vi "ProcessActiveMeasurements.vi"(1 "Active Measurements":T1[](array[typedef])) -> (0 "Measurements":T5)   [LabVIEW 2025]
uses:
  NewCurveDataEventArgs.ctl
  E:/PSCode/PalmSens_SDK/labview/PalmSens/Libraries/PalmSens.Core.Simplified.LabVIEW.dll
  Libraries/PalmSens.Core.Simplified.LabVIEW.dll
  LiveCurveResult.ctl
  MeasurementsResult.ctl
  MeasurementResults.ctl
  CurvesByMeasurement.ctl
  MeasurementInfo.ctl
  CurveInfo.ctl
  MeasurementEventArgs.ctl
  ActiveCurve.ctl
  ActiveMeasurementInfo.ctl
panel:
  out "Processing Completed Event":refnum<user-event>
  out "Active Curve Event":refnum<user-event>
  out "Active Measurement Event":refnum<user-event>
  out "Curves By Measurement":T2
  out "Active Measurement":refnum<k24>
  out "New Curve Values":T8
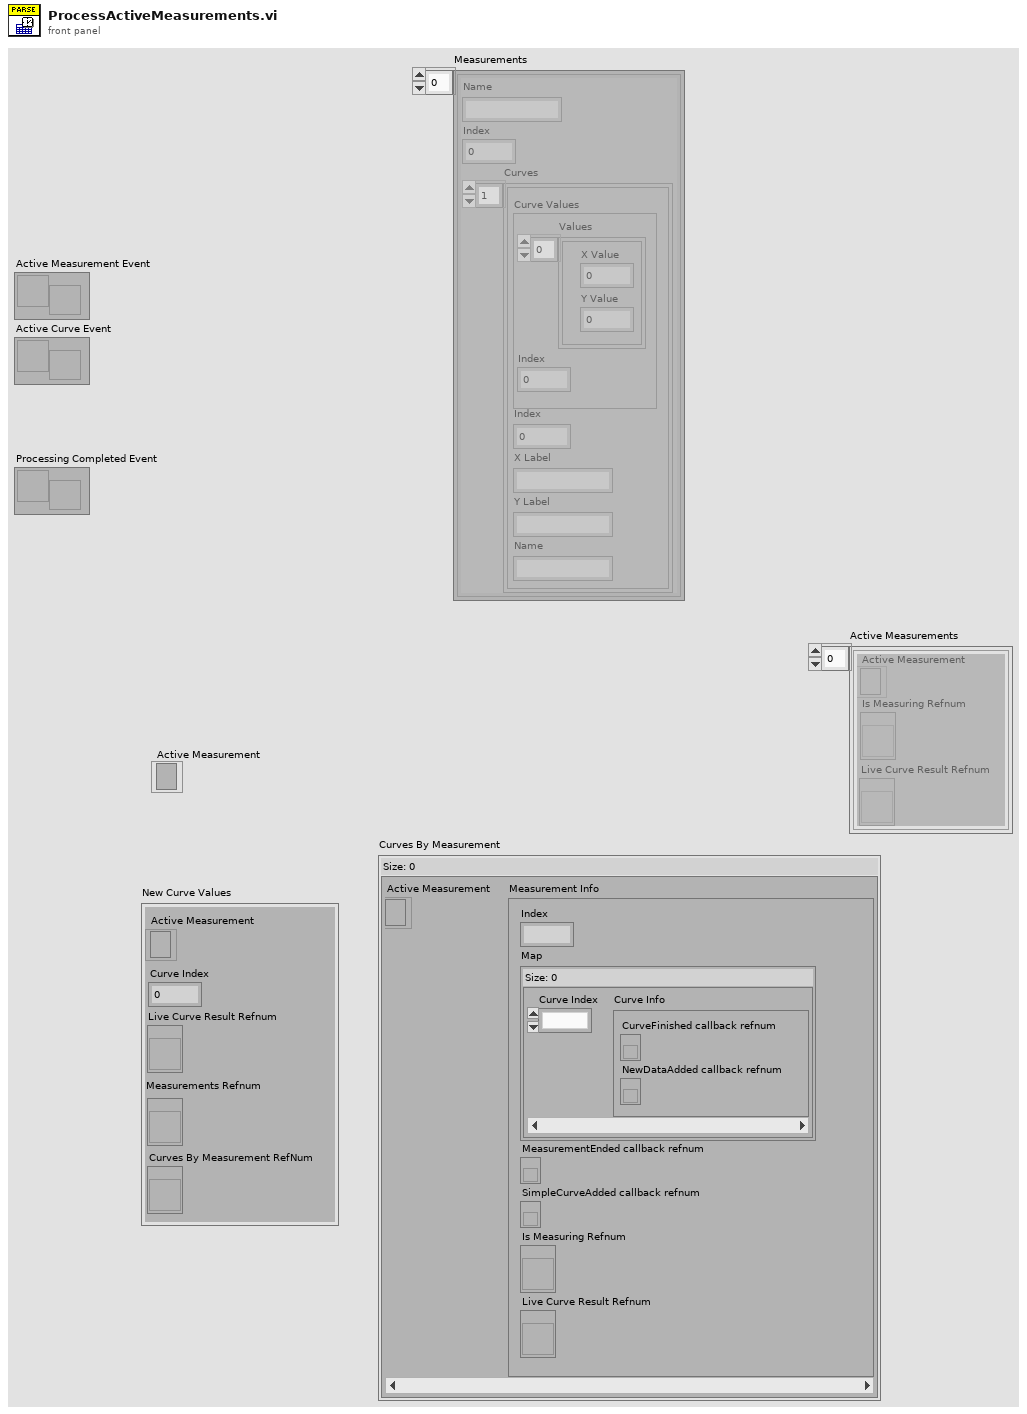
[diagram p1: front panel]
types:
  T1 = typedef "ActiveMeasurementInfo.ctl" = cluster{"Active Measurement":refnum<k24>, "Is Measuring Refnum":refnum<vi>, "Live Curve Result Refnum":refnum<vi>}
  T2 = typedef "CurvesByMeasurement.ctl" = map{refnum<k24>, T3}
  T3 = typedef "MeasurementInfo.ctl" = cluster{"Index":i32, "Is Measuring Refnum":refnum<vi>, "MeasurementEnded callback refnum":refnum<k27>, "SimpleCurveAdded callback refnum":refnum<k27>, "Live Curve Result Refnum":refnum<vi>, "Map":map{i32, T4}}
  T4 = typedef "CurveInfo.ctl" = cluster{"NewDataAdded callback refnum":refnum<k27>, "CurveFinished callback refnum":refnum<k27>}
  T5 = typedef "MeasurementsResult.ctl" = cluster{"Name":string, "Curves":T6, "Index":i32}[]
  T6 = typedef "MeasurementResults.ctl" = T7[]
  T7 = typedef "LiveCurveResult.ctl" = cluster{"X Label":string, "Y Label":string, "Name":string, "Index":i16, "Curve Values":cluster{"Values":cluster{"X Value":dbl, "Y Value":dbl}[], "Index":i16}}
  T8 = typedef "NewCurveDataEventArgs.ctl" = cluster{"Active Measurement":refnum<k24>, "Live Curve Result Refnum":refnum<vi>, "Measurements Refnum":refnum<vi>, "Curves By Measurement RefNum":refnum<vi>, "Curve Index":i32}
  T9 = typedef "ActiveCurve.ctl" = cluster{"Active Measurement":refnum<k24>, "Dispose":bool, "Curve Index":i32}
  T10 = typedef "MeasurementEventArgs.ctl" = cluster{"Active Measurement":refnum<k24>, "Dispose":bool}
  T11 = cluster{"Active Curve":T9, "Active Curve Event":refnum<user-event>}
  T12 = cluster{"Active Measurement":refnum<k24>, "Active Measurement Event":refnum<user-event>}
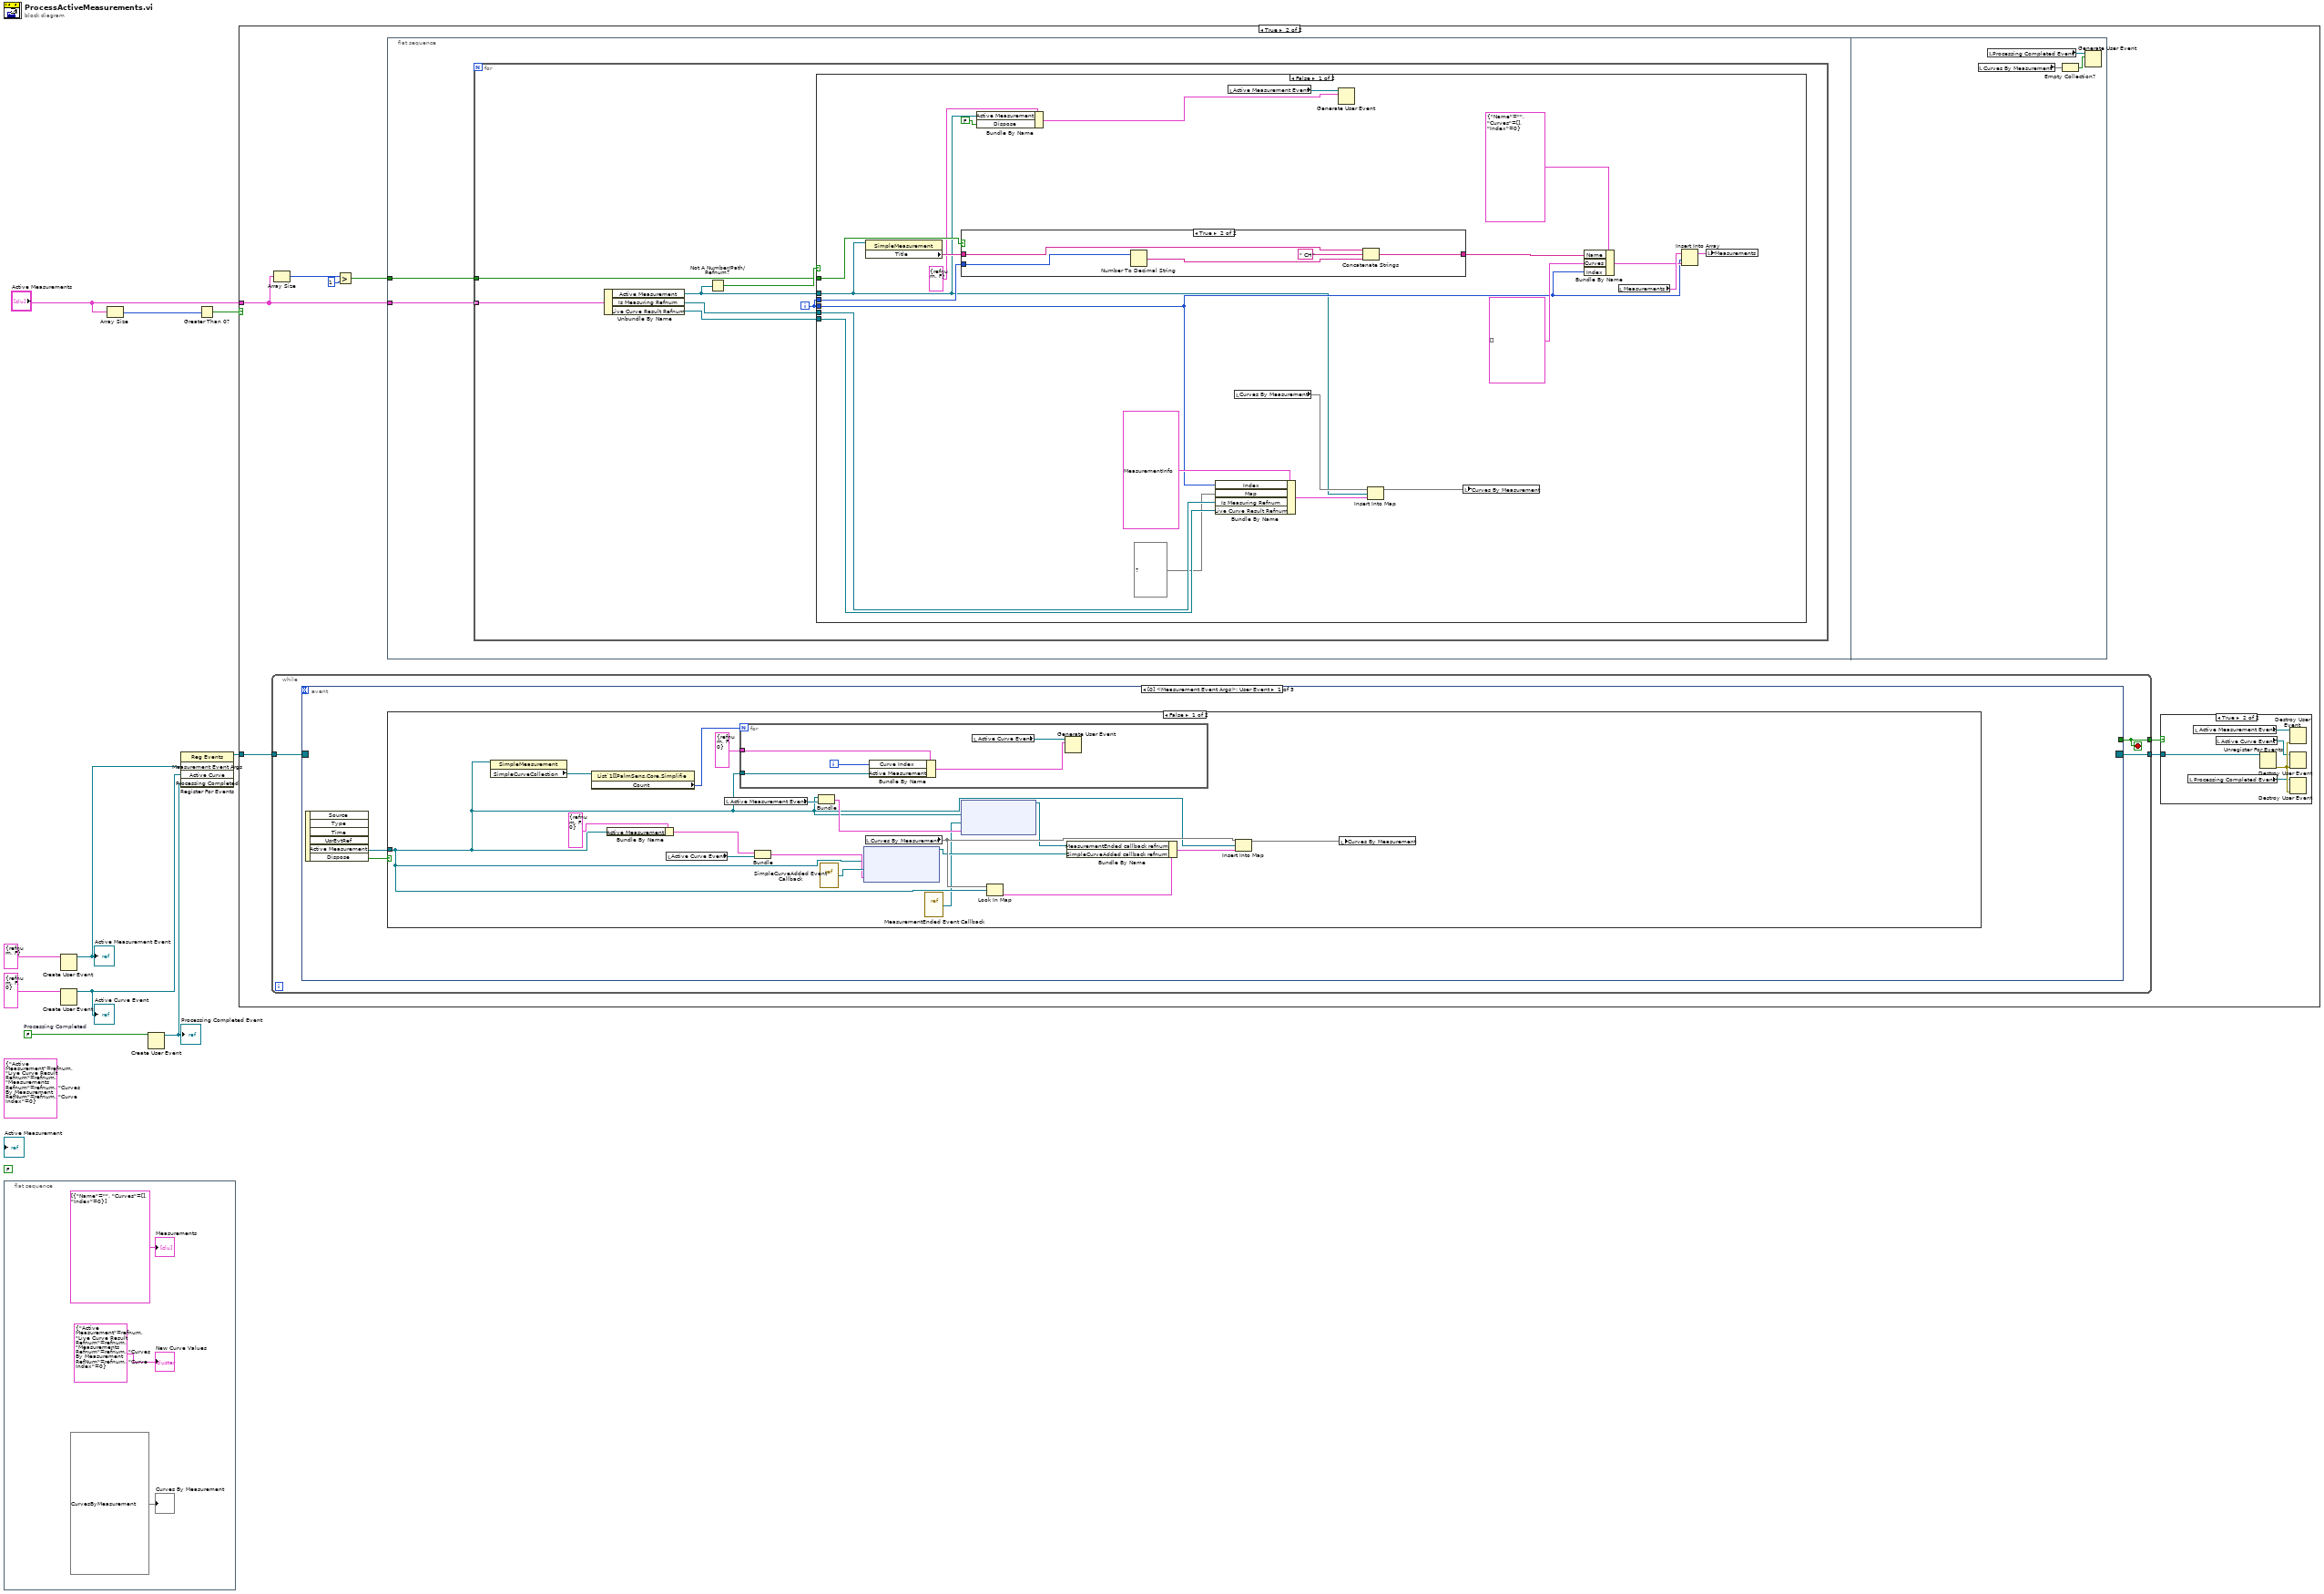
[diagram p0: block diagram]
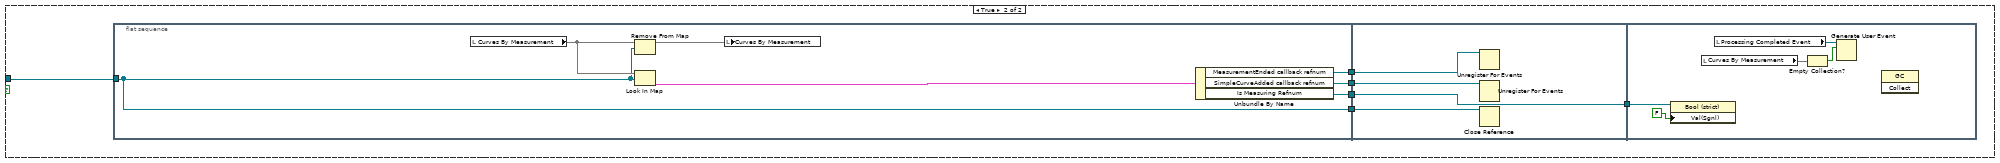
[diagram p4: hidden frame]
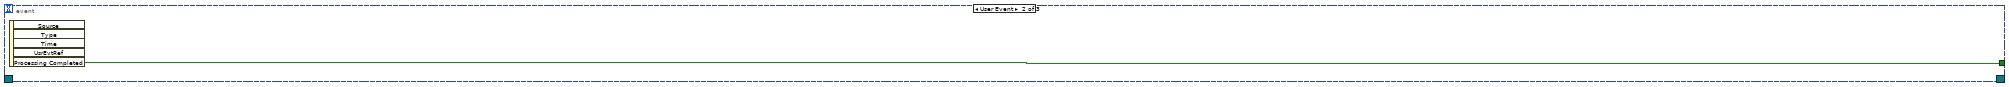
[diagram p5: hidden frame]
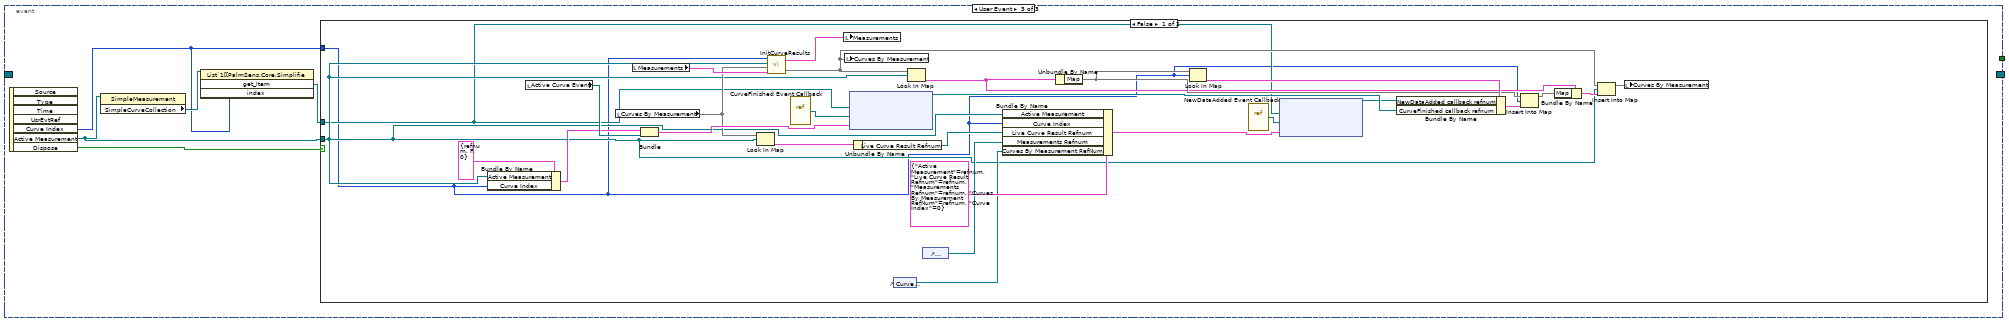
[diagram p6: hidden frame]
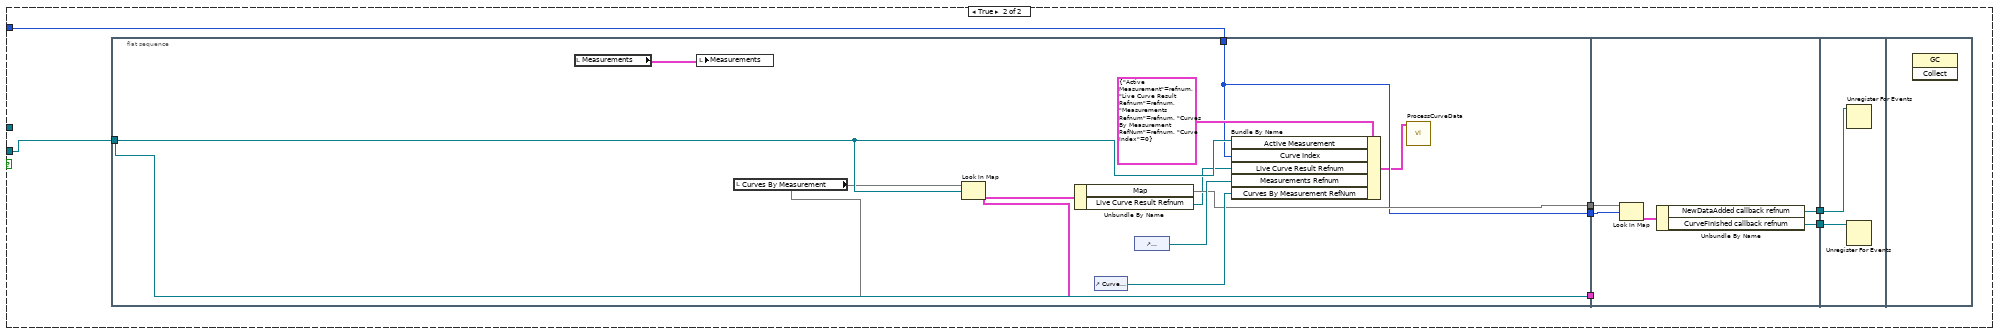
[diagram p7: hidden frame]
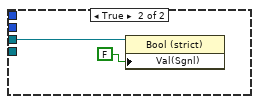
[diagram p9: hidden frame]
diagram:
  w5 = FALSE  # Processing Completed
  (unwired) T8 {"Active Measurement"=refnum, "Live Curve Result Refnum"=refnum, "Measurements Refnum"=refnum, "Curves By Measurement RefNum"=refnum, "Curve Index"=0} ("New Curve Values")
  (unwired) FALSE ("Processing Completed")
  n1 = flat-sequence {
    frame #0 {
      "New Curve Values" <- T8 {"Active Measurement"=refnum, "Live Curve Result Refnum"=refnum, "Measurements Refnum"=refnum, "Curves By Measurement RefNum"=refnum, "Curve Index"=0} ("New Curve Values")
      "Measurements" <- T5 [{"Name"="", "Curves"=[], "Index"=0}] ("Measurements")
      "Curves By Measurement" <- T2 {} ("Curves By Measurement")
    }
  }
  n2 = Create User Event(user event datatype=T10 {"Active Measurement"=refnum, "Dispose"=FALSE} ("Measurement Event Args")) -> (user event=w4:refnum<user-event>)  [unwired: 1 in, 1 out]
  "Active Measurement Event" <- w4
  n3 = Create User Event(user event datatype=T9 {"Active Measurement"=refnum, "Dispose"=FALSE, "Curve Index"=0} ("Active Curve")) -> (user event=w3:refnum<user-event>)  [unwired: 1 in, 1 out]
  "Active Curve Event" <- w3
  n4 = Array Size(array="Active Measurements") -> (size(s)=w10:i32)
  n5 = Create User Event(user event datatype=w5) -> (user event=w2:refnum<user-event>)  [unwired: 1 in, 1 out]
  "Processing Completed Event" <- w2
  n6 = register-events(w4, w3, w2) -> (reference out=w7:refnum<event-registration>)  [unwired: 2 in, 1 out]
  n7 = Greater Than 0?(x=w10) -> (x > 0?=w9:bool)
  n8 = case shown="True" w9 {
    tunnel: "Active Measurements" -> [_ w18]
    tunnel: w7 -> [_ w16]
    frame False {
    }
    frame True {
      n9 = while {
        tunnel: w16 -> [w27]
        tunnel: [w28] -> w15
        tunnel: [w26] -> w14
        stop <- w26 stop-if-true
        n10 = event shown="[0] <Measurement Event Args>: User Event" {
          selector: w27 -> [_ _ _]
          dyn-events: [_ _ _] -> w28
          timeout: _ -> [_ _ _]
          tunnel: [_ w76 _] -> w26
          event User Event {
            n11 = event-data() -> ("Active Measurement"=w30:refnum<k24>, "Dispose"=w29:bool)  [unwired: 1 in, 4 out]
            n12 = case shown="False" w29 {
              tunnel: w30 -> [w32 w54]
              frame False {
                n13 = property class="SimpleMeasurement"(reference=w32) -> ("SimpleCurveCollection"=w42:refnum<k24>)  [unwired: 1 in, 2 out]
                n14 = property class="List`1[[PalmSens.Core.Simplifie"(reference=w42) -> ("Count"=w43:i32)  [unwired: 1 in, 2 out]
                n15 = Bundle By Name(cluster=T9 {"Active Measurement"=refnum, "Dispose"=FALSE, "Curve Index"=0} ("Active Curve"), "Active Measurement"=w32) -> (w46:T9)
                n16 = local read "Active Curve Event"() -> (w45:refnum<user-event>)
                n17 = local read "Active Measurement Event"() -> (w44:refnum<user-event>)
                n18 = for {
                  N: w43 -> [_]
                  tunnel: T9 {"Active Measurement"=refnum, "Dispose"=FALSE, "Curve Index"=0} ("Active Curve") -> [w53]
                  tunnel: w32 -> [w52]
                  i -> [w49]
                  n19 = Bundle By Name(cluster=w53, "Curve Index"=w49, "Active Measurement"=w52) -> (w51:T9)
                  n20 = local read "Active Curve Event"() -> (w50:refnum<user-event>)
                  n21 = Generate User Event(user event=w50, event data cluster=w51) -> ()  [unwired: 2 in, 2 out]
                }
                n22 = Bundle("Active Curve"=w46, "Active Curve Event"=w45) -> (w47:T11)  [unwired: 1 in]
                n23 = Bundle("Active Measurement"=w32, "Active Measurement Event"=w44) -> (w35:T12)  [unwired: 1 in]
                n24 = vi-ref "SimpleCurveAdded Event Callback.vi"() -> ("vi reference"=w48:refnum<vi>)
                n25 = node(w32, w48, w47) -> (w36:refnum<k27>)  [unwired: 2 in, 1 out]
                n26 = local read "Curves By Measurement"() -> (w40:T2)
                n27 = vi-ref "MeasurementEnded Event Callback.vi"() -> ("vi reference"=w31:refnum<vi>)
                n28 = node(w32, w31, w35) -> (w37:refnum<k27>)  [unwired: 2 in, 1 out]
                n29 = Look In Map(map=w40, key=w32) -> (value=w39:T3)  [unwired: 1 in, 1 out]
                n30 = Bundle By Name(cluster=w39, "MeasurementEnded callback refnum"=w37, "SimpleCurveAdded callback refnum"=w36) -> (w38:T3)
                n31 = Insert Into Map(map in=w40, key=w32, value=w38) -> (map out=w41:T2)  [unwired: 2 out]
                n32 = local write "Curves By Measurement"(w41) -> ()
              }
              frame True {
                n33 = flat-sequence {
                  tunnel: w54 -> [w64]
                  tunnel: [w64] -> w59
                  tunnel: [w62] -> w58
                  tunnel: [w61] -> w57
                  tunnel: [w60] -> w56
                  tunnel: w59 -> [w69]
                  tunnel: w58 -> [w68]
                  tunnel: w57 -> [w67]
                  tunnel: [w70] -> w55
                  tunnel: w56 -> [w70]
                  tunnel: w55 -> [w73]
                  frame #0 {
                    n34 = local read "Curves By Measurement"() -> (w65:T2)
                    n35 = Remove From Map(10:w64, 11:w65) -> (3:w63:T2)  [unwired: 2 out]
                    n36 = Look In Map(map=w65, key=w64) -> (value=w66:T3)  [unwired: 1 in, 1 out]
                    n37 = local write "Curves By Measurement"(w63) -> ()
                    n38 = Unbundle By Name(w66) -> ("MeasurementEnded callback refnum"=w62:refnum<k27>, "SimpleCurveAdded callback refnum"=w61:refnum<k27>, "Is Measuring Refnum"=w60:refnum<vi>)
                  }
                  frame #1 {
                    n39 = Unregister For Events(event registration refnum=w68) -> ()  [unwired: 1 in, 1 out]
                    n40 = Unregister For Events(event registration refnum=w67) -> ()  [unwired: 1 in, 1 out]
                    n41 = Close Reference(reference=w69) -> ()  [unwired: 1 in, 1 out]
                  }
                  frame #2 {
                    n42 = property class="Bool (strict)"(reference=w73, "Val(Sgnl)"=FALSE ("Value (Signaling)")) -> ()  [unwired: 1 in, 2 out]
                    n43 = local read "Curves By Measurement"() -> (w74:T2)
                    n44 = local read "Processing Completed Event"() -> (w72:refnum<user-event>)
                    n45 = Empty Collection?(1:w74) -> (0:w71:bool)
                    n46 = Generate User Event(user event=w72, event data cluster=w71) -> ()  [unwired: 2 in, 2 out]
                    n47 = invoke class="GC" method="Collect"() -> ()  [unwired: 3 in, 3 out]
                  }
                }
              }
            }
          }
          event User Event {
            n48 = event-data() -> ("Processing Completed"=w76:bool)  [unwired: 1 in, 4 out]
          }
          event User Event {
            n49 = event-data() -> ("Curve Index"=w78:i32, "Active Measurement"=w80:refnum<k24>, "Dispose"=w81:bool)  [unwired: 1 in, 4 out]
            n50 = property class="SimpleMeasurement"(reference=w80) -> ("SimpleCurveCollection"=w79:refnum<k24>)  [unwired: 1 in, 2 out]
            n51 = invoke class="List`1[[PalmSens.Core.Simplifie" method="get_Item"(reference=w79, "index"=w78) -> ("get_Item"=w77:refnum<k24>)  [unwired: 2 in, 3 out]
            n52 = case shown="False" w81 {
              tunnel: w77 -> [w83 _]
              tunnel: w80 -> [w84 w112]
              tunnel: w78 -> [w82 w111]
              frame False {
                n53 = Bundle By Name(cluster=T9 {"Active Measurement"=refnum, "Dispose"=FALSE, "Curve Index"=0} ("Active Curve"), "Active Measurement"=w84, "Curve Index"=w82) -> (w107:T9)
                n54 = local read "Active Curve Event"() -> (w109:refnum<user-event>)
                n55 = local read "Curves By Measurement"() -> (w89:T2)
                n56 = local read "Measurements"() -> (w93:T5)
                n57 = Bundle("Active Curve"=w107, "Active Curve Event"=w109) -> (w106:T11)  [unwired: 1 in]
                n58 = Look In Map(map=w89, key=w84) -> (value=w88:T3)  [unwired: 1 in, 1 out]
                n59 = call "InitCurveResults.vi"("Measurements In"=w93, "Curves By Measurement In"=w89, "Active Measurement"=w84, "Curve Index"=w82) -> ("Curves By Measurement Out"=w95:T2, "Measurements Out"=w94:T5)
                n60 = vi-ref "CurveFinished Event Callback.vi"() -> ("vi reference"=w105:refnum<vi>)
                n61 = local write "Measurements"(w94) -> ()
                n62 = local write "Curves By Measurement"(w95) -> ()
                n63 = node(w83, w105, w106) -> (w102:refnum<k27>)  [unwired: 2 in, 1 out]
                n64 = Unbundle By Name(w88) -> ("Live Curve Result Refnum"=w87:refnum<vi>)
                n65 = control-ref of="Curves By Measurement"() -> (w86:refnum<vi>)
                n66 = Look In Map(map=w95, key=w84) -> (value=w98:T3)  [unwired: 1 in, 1 out]
                n67 = control-ref of="Measurements"() -> (w92:refnum<vi>)
                n68 = Bundle By Name(cluster=T8 {"Active Measurement"=refnum, "Live Curve Result Refnum"=refnum, "Measurements Refnum"=refnum, "Curves By Measurement RefNum"=refnum, "Curve Index"=0} ("New Curve Values"), "Active Measurement"=w84, "Curve Index"=w82, "Live Curve Result Refnum"=w87, "Measurements Refnum"=w92, "Curves By Measurement RefNum"=w86) -> (w91:T8)
                n69 = Unbundle By Name(w98) -> ("Map"=w99:map{i32, T4})
                n70 = Look In Map(map=w99, key=w82) -> (value=w103:T4)  [unwired: 1 in, 1 out]
                n71 = vi-ref "NewDataAdded Event Callback.vi"() -> ("vi reference"=w90:refnum<vi>)
                n72 = node(w83, w90, w91) -> (w101:refnum<k27>)  [unwired: 2 in, 1 out]
                n73 = Bundle By Name(cluster=w103, "NewDataAdded callback refnum"=w101, "CurveFinished callback refnum"=w102) -> (w100:T4)
                n74 = Insert Into Map(map in=w99, key=w82, value=w100) -> (map out=w97:map{i32, T4})  [unwired: 2 out]
                n75 = Bundle By Name(cluster=w98, "Map"=w97) -> (w96:T3)
                n76 = Insert Into Map(map in=w95, key=w84, value=w96) -> (map out=w85:T2)  [unwired: 2 out]
                n77 = local write "Curves By Measurement"(w85) -> ()
              }
              frame True {
                n78 = flat-sequence {
                  tunnel: w112 -> [w128]
                  tunnel: [w128] -> w118
                  tunnel: [w125] -> w117
                  tunnel: [w124] -> w116
                  tunnel: [w123] -> w115
                  tunnel: w111 -> [w120]
                  tunnel: [w120] -> w110
                  tunnel: [w133] -> w114
                  tunnel: [w132] -> w113
                  tunnel: w118 -> [_]
                  tunnel: w117 -> [_]
                  tunnel: w116 -> [_]
                  tunnel: w115 -> [w131]
                  tunnel: w110 -> [w130]
                  tunnel: w114 -> [w136]
                  tunnel: w113 -> [w135]
                  frame #0 {
                    n79 = local read "Measurements"() -> (w121:T5)
                    n80 = local write "Measurements"(w121) -> ()
                    n81 = local read "Curves By Measurement"() -> (w125:T2)
                    n82 = Look In Map(map=w125, key=w128) -> (value=w124:T3)  [unwired: 1 in, 1 out]
                    n83 = Unbundle By Name(w124) -> ("Map"=w123:map{i32, T4}, "Live Curve Result Refnum"=w122:refnum<vi>)
                    n84 = control-ref of="Curves By Measurement"() -> (w126:refnum<vi>)
                    n85 = control-ref of="Measurements"() -> (w127:refnum<vi>)
                    n86 = Bundle By Name(cluster=T8 {"Active Measurement"=refnum, "Live Curve Result Refnum"=refnum, "Measurements Refnum"=refnum, "Curves By Measurement RefNum"=refnum, "Curve Index"=0} ("New Curve Values"), "Active Measurement"=w128, "Curve Index"=w120, "Live Curve Result Refnum"=w122, "Measurements Refnum"=w127, "Curves By Measurement RefNum"=w126) -> (w119:T8)
                    n87 = call "ProcessCurveData.vi"("New Curve Values"=w119) -> ()  [unwired: 11 in]
                  }
                  frame #1 {
                    n88 = Look In Map(map=w131, key=w130) -> (value=w134:T4)  [unwired: 1 in, 1 out]
                    n89 = Unbundle By Name(w134) -> ("NewDataAdded callback refnum"=w133:refnum<k27>, "CurveFinished callback refnum"=w132:refnum<k27>)
                  }
                  frame #2 {
                    n90 = Unregister For Events(event registration refnum=w136) -> ()  [unwired: 1 in, 1 out]
                    n91 = Unregister For Events(event registration refnum=w135) -> ()  [unwired: 1 in, 1 out]
                  }
                  frame #3 {
                    n92 = invoke class="GC" method="Collect"() -> ()  [unwired: 3 in, 3 out]
                  }
                }
              }
            }
          }
        }
      }
      n93 = Array Size(array=w18) -> (size(s)=w20:i32)
      n94 = Greater?(x=w20, y=1) -> (0:w17:bool)
      n95 = flat-sequence {
        tunnel: w18 -> [w138]
        tunnel: w17 -> [w137]
        frame #0 {
          n96 = for {
            tunnel: w138 -> [w145] mode=indexing
            tunnel: w137 -> [w140]
            i -> [w141]
            n97 = Unbundle By Name(w145) -> ("Active Measurement"=w143:refnum<k24>, "Is Measuring Refnum"=w142:refnum<vi>, "Live Curve Result Refnum"=w139:refnum<vi>)
            n98 = Not A Number/Path/Refnum?(number/path/refnum=w143) -> (NaN/Path/Refnum?=w144:bool)
            n99 = case shown="False" w144 {
              tunnel: w141 -> [w158 _]
              tunnel: w143 -> [w150 _]
              tunnel: w142 -> [w157 w175]
              tunnel: w141 -> [w156 _]
              tunnel: w140 -> [w153 _]
              tunnel: w139 -> [w147 _]
              frame False {
                n100 = property class="SimpleMeasurement"(reference=w150) -> ("Title"=w155:string)  [unwired: 1 in, 2 out]
                n101 = case shown="True" w153 {
                  tunnel: w155 -> [w168 w173]
                  tunnel: w156 -> [_ w171]
                  tunnel: [w168 w169] -> w154
                  frame False {
                  }
                  frame True {
                    n102 = Number To Decimal String(number=w171) -> (decimal integer string=w170:string)  [unwired: 1 in]
                    n103 = Concatenate Strings(w173, " CH" ("string"), w170) -> (w169:string)
                  }
                }
                n104 = Bundle By Name(cluster=T10 {"Active Measurement"=refnum, "Dispose"=FALSE} ("Measurement Event Args"), "Active Measurement"=w150, "Dispose"=FALSE) -> (w149:T10)
                n105 = Bundle By Name(cluster=T3 {"Index"=0, "Is Measuring Refnum"=refnum, "MeasurementEnded callback refnum"=refnum, "SimpleCurveAdded callback refnum"=refnum, "Live Curve Result Refnum"=refnum, "Map"={}} ("Measurement Info"), "Index"=w158, "Map"=map{i32, T4} {}, "Is Measuring Refnum"=w157, "Live Curve Result Refnum"=w147) -> (w165:T3)
                n106 = local read "Active Measurement Event"() -> (w148:refnum<user-event>)
                n107 = local read "Curves By Measurement"() -> (w167:T2)
                n108 = Generate User Event(user event=w148, event data cluster=w149) -> ()  [unwired: 2 in, 2 out]
                n109 = Insert Into Map(map in=w167, key=w150, value=w165) -> (map out=w166:T2)  [unwired: 2 out]
                n110 = local write "Curves By Measurement"(w166) -> ()
                n111 = Bundle By Name(cluster=cluster{"Name":string, "Curves":T6, "Index":i32} {"Name"="", "Curves"=[], "Index"=0} ("new element/subarray"), "Name"=w154, "Curves"=T6 [], "Index"=w158) -> (w161:cluster{"Name":string, "Curves":T6, "Index":i32})
                n112 = local read "Measurements"() -> (w163:T5)
                n113 = Insert Into Array(array=w163, index=w158, new element=w161) -> (w162:T5)
                n114 = local write "Measurements"(w162) -> ()
              }
              frame True {
                n115 = property class="Bool (strict)"(reference=w175, "Val(Sgnl)"=FALSE ("Value (Signaling)")) -> ()  [unwired: 1 in, 2 out]
              }
            }
          }
        }
        frame #1 {
          n116 = local read "Curves By Measurement"() -> (w178:T2)
          n117 = local read "Processing Completed Event"() -> (w176:refnum<user-event>)
          n118 = Empty Collection?(1:w178) -> (0:w177:bool)
          n119 = Generate User Event(user event=w176, event data cluster=w177) -> ()  [unwired: 2 in, 2 out]
        }
      }
      n120 = case shown="True" w14 {
        tunnel: w15 -> [_ w25]
        frame False {
        }
        frame True {
          n121 = local read "Processing Completed Event"() -> (w21:refnum<user-event>)
          n122 = local read "Active Measurement Event"() -> (w24:refnum<user-event>)
          n123 = local read "Active Curve Event"() -> (w22:refnum<user-event>)
          n124 = Unregister For Events(event registration refnum=w25) -> (error out=w23:errorcluster)  [unwired: 1 in]
          n125 = Destroy User Event(user event=w24, error in=w23) -> ()  [unwired: 1 out]
          n126 = Destroy User Event(user event=w22, error in=w23) -> ()  [unwired: 1 out]
          n127 = Destroy User Event(user event=w21, error in=w23) -> ()  [unwired: 1 out]
        }
      }
    }
  }
